vi "save_data.vi"(6 "wl-current array":dbl[][](array[numeric]) caption="Data array", 7 "Application Directory":string, 11 "Filepath in":path) -> (3 "Filepath out":path)   [LabVIEW 2018]
uses:
  <vilib>/Utility/file.llb/Write Delimited Spreadsheet (DBL).vi
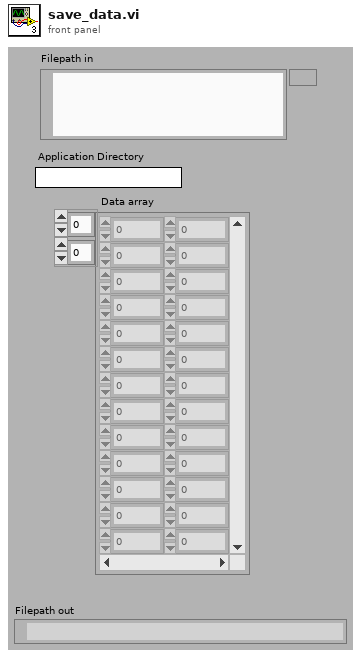
[diagram p1: front panel]
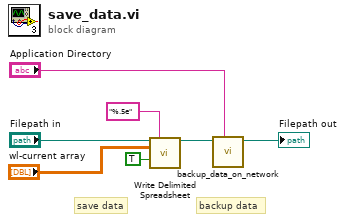
[diagram p0: block diagram]
diagram:
  # "backup data"
  # "save data"
  n1 = call-poly <vilib>:"Write Delimited Spreadsheet.vi"("file path (dialog if empty)"="Filepath in", "format (%.3f)"="%.5e", "2D data"="wl-current array", "append to file? (new file:F)"=TRUE) -> ("new file path (Not A Path if cancelled)"=w7:path)  [unwired: 10 in, 1 out]
  n2 = call "backup_data_on_network.vi"("Application Directory"="Application Directory", "Filepath in"=w7) -> ("Filepath out"=→"Filepath out":path)  [unwired: 9 in]
